vi "Set Phase Angle.vi"(8 "error in (no error)":errorcluster, 9 "Phase Angle (T: Lead)":bool=TRUE, 10 "Phase Angle Value (0.0)":dbl min=0.0 max=1.0 format="%.3f", 11 "VISA resource name":refnum<visa-resource-name>) -> (0 "error out":errorcluster, 3 "VISA resource name out":refnum<visa-resource-name>)   [LabVIEW 2011, in "Fluke 5XXX Series Multicalibrators.lvlib"]
doc: "This VI sets the diplacement power factor (phase angle) between the calibrator front panel terminals NORMAL and AUX (for sinewaves output only). The NORMAL terminal output is the phase reference.\n\nNote:\n\nThis VI is available only for instrument models 5500A and 5520A."
uses:
  Fluke 5XXX Series Multicalibrators.lvlib
panel:
  # "Lead"
  # "Lag"
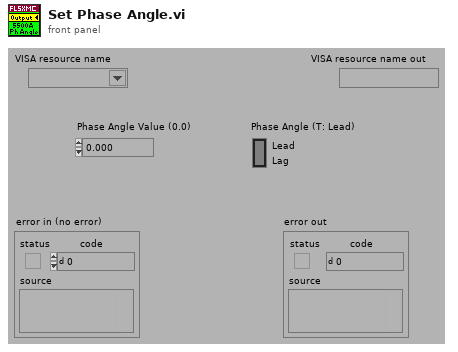
[diagram p1: front panel]
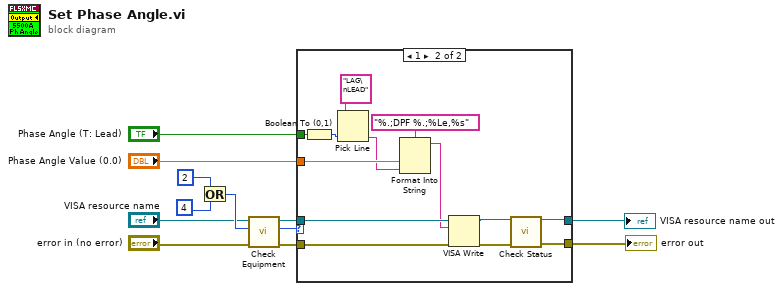
[diagram p0: block diagram]
diagram:
  n1 = Or(x=2 ("Numeric"), y=4 ("Numeric")) -> (x .or. y?=w9:i32)
  n2 = call "Check Equipment.vi"("error in (no error)"="error in (no error)", "Bit Mask"=w9, "VISA resource name"="VISA resource name") -> ("error out"=w12:errorcluster, "Present?"=w11:u32, "VISA resource name out"=w10:refnum<visa-resource-name>)  [unwired: 6 in]
  n3 = case shown="1" w11 {
    tunnel: [w13 w22] -> w4
    tunnel: w12 -> [w14 w27]
    tunnel: w10 -> [w13 w26]
    tunnel: [w14 w25] -> w3
    tunnel: "Phase Angle (T: Lead)" -> [_ w19]
    tunnel: "Phase Angle Value (0.0)" -> [_ w18]
    frame 0, Default {
    }
    frame 1 {
      n4 = Boolean To (0,1)(Boolean=w19) -> (0, 1=w16:i16)
      n5 = Pick Line(multi-line string="LAG\nLEAD", line index=w16) -> (output string=w17:string)  [unwired: 1 in]
      n6 = Format Into String(format string="%.;DPF %.;%Le,%s", w18, w17) -> (resulting string=w20:string)  [unwired: 2 in, 1 out]
      n7 = VISA Write(VISA resource name=w26, write buffer=w20, error in (no error)=w27) -> (VISA resource name out=w23:refnum<visa-resource-name>, error out=w24:errorcluster)  [unwired: 1 out]
      n8 = call "Check Status.vi"("VISA resource name"=w23, "error in (no error)"=w24) -> ("VISA resource name out"=w22:refnum<visa-resource-name>, "error out"=w25:errorcluster)  [unwired: 12 in]
    }
  }
  "VISA resource name out" <- w4
  "error out" <- w3
